vi "ArchiveinPlace Value Change.vi"(7 "Control Refs":T1, 9 "Linux?":bool, 10 "archive in place":bool caption="Archive Old Logs in Original Directory", 11 "References":T2) -> (0 "error out":errorcluster)   [LabVIEW 2015, in "TDMS datalogger editor node.lvclass"]
uses:
  TDMS datalogger editor node.lvclass
  <vilib>/NI/DCAF/Tag Editor Core/Table API/Table Manager/object ref.ctl
  <vilib>/NI/DCAF/Tag Editor Core/Configuration Editor/Classes/Engine Parent/Engine Parent Editor Node.lvclass
  <vilib>/NI/DCAF/Tag Editor Core/Configuration Editor/Classes/Module editor node/module editor node.lvclass
  Control Refs.ctl
  TDMS datalogger editor node.lvclass/TDMS datalogger editor node.ctl
  module/configuration/TDMS datalogger configuration.lvclass/TDMS datalogger configuration.ctl
  module/configuration/Read logrotate_options.vi
  module/configuration/Write logrotate_options.vi
  module/configuration/TDMS datalogger configuration.lvclass
  <vilib>/NI/DCAF/Tag Editor Core/Table API/Table Manager/Table Manager.lvclass
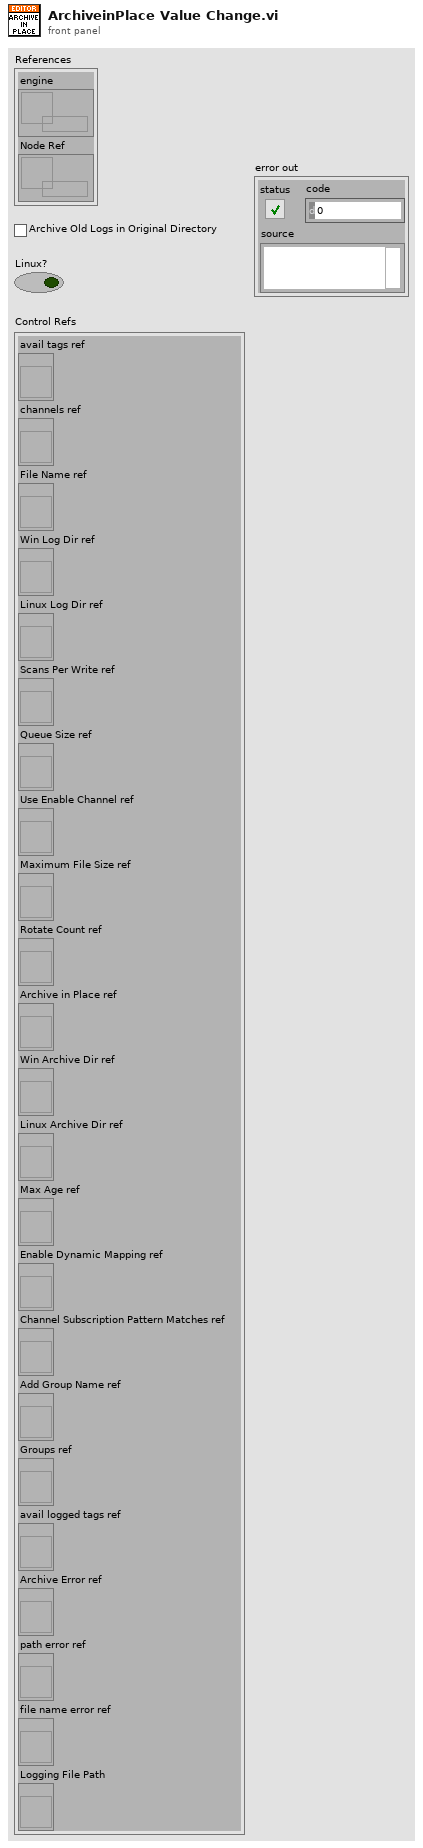
[diagram p1: front panel]
types:
  T1 = typedef "Control Refs.ctl" = cluster{"avail tags ref":refnum<vi>, "channels ref":refnum<vi>, "File Name ref":refnum<vi>, "Win Log Dir ref":refnum<vi>, "Linux Log Dir ref":refnum<vi>, "Scans Per Write ref":refnum<vi>, "Queue Size ref":refnum<vi>, "Use Enable Channel ref":refnum<vi>, "Maximum File Size ref":refnum<vi>, "Rotate Count ref":refnum<vi>, "Archive in Place ref":refnum<vi>, "Win Archive Dir ref":refnum<vi>, "Linux Archive Dir ref":refnum<vi>, "Max Age ref":refnum<vi>, "Enable Dynamic Mapping ref":refnum<vi>, "Channel Subscription Pattern Matches ref":refnum<vi>, "Add Group Name ref":refnum<vi>, "Groups ref":refnum<vi>, "avail logged tags ref":refnum<vi>, "Archive Error ref":refnum<vi>, "path error ref":refnum<vi>, "file name error ref":refnum<vi>, "Logging File Path":refnum<vi>}
  T2 = typedef "Table Manager.lvlib/Table Manager.lvclass/object ref.ctl" = cluster{"engine":refnum<data-value>, "Node Ref":refnum<data-value>}
  T3 = typedef "LogRotate.lvclass/options.ctl" = cluster{"max file size (bytes)":i64, "rotate count":u32, "max age (days)":dbl, "No archive dir":bool, "Archive dir":path}
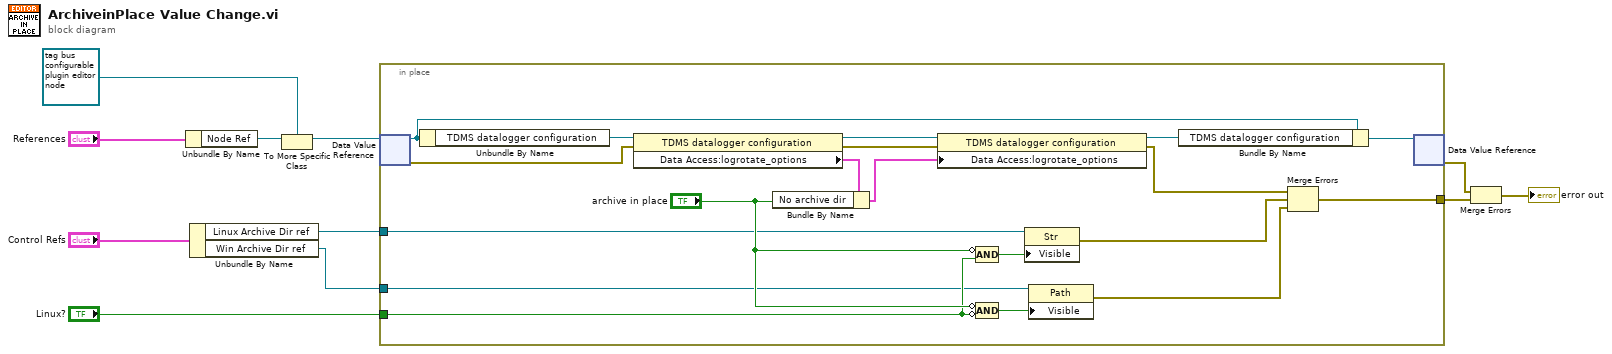
[diagram p0: block diagram]
diagram:
  n1 = Unbundle By Name("References") -> ("Node Ref"=w10:refnum<data-value>)
  n2 = Unbundle By Name("Control Refs") -> ("Linux Archive Dir ref"=w2:refnum<vi>, "Win Archive Dir ref"=w1:refnum<vi>)
  n3 = To More Specific Class(target class=refnum<data-value> refnum ("data value reference"), reference=w10) -> (specific class reference=w8:refnum<data-value>)  [unwired: 1 in, 1 out]
  n4 = in-place {
    in-place-border: [w16] -> w6
    in-place-border: "Linux?" -> [w18]
    in-place-border: w2 -> [w13]
    in-place-border: w1 -> [w12]
    n5 = in-place-dvr #1(w8) -> (w25:refnum<class "TDMS datalogger editor node.lvclass">, w17:errorcluster)
    n6 = Unbundle By Name(w25) -> ("TDMS datalogger configuration"=w30:refnum<class "TDMS datalogger configuration.lvclass">)
    n7 = property class="TDMS datalogger configuration"(reference=w30, error in=w17) -> (reference out=w28:refnum<class "TDMS datalogger configuration.lvclass">, error out=w27:errorcluster, "Data Access:logrotate_options"=w29:T3)
    n8 = Bundle By Name(cluster=w29, "No archive dir"="archive in place") -> (w26:T3)
    n9 = property class="TDMS datalogger configuration"(reference=w28, error in=w27, "Data Access:logrotate_options"=w26) -> (reference out=w24:refnum<class "TDMS datalogger configuration.lvclass">, error out=w22:errorcluster)
    n10 = Compound Arithmetic op=AND(invert "archive in place", w18) -> (w21:bool)
    n11 = Compound Arithmetic op=AND(invert "archive in place", invert w18) -> (w20:bool)
    n12 = property on="Property Node" class="Str"(reference=w13, "Visible"=w21) -> (error out=w15:errorcluster)  [unwired: 1 in, 1 out]
    n13 = property on="Property Node" class="Path"(reference=w12, "Visible"=w20) -> (error out=w14:errorcluster)  [unwired: 1 in, 1 out]
    n14 = Bundle By Name(cluster=w25, "TDMS datalogger configuration"=w24) -> (w23:refnum<class "TDMS datalogger editor node.lvclass">)
    n15 = Merge Errors(w22, w15, w14) -> (w16:errorcluster)
    n16 = in-place-dvr #1(w23) -> (w4:errorcluster)  [unwired: 1 out]
  }
  n17 = Merge Errors(w4, w6) -> (→"error out":errorcluster)
